vi "Test Tree.vi"() -> ()   [LabVIEW 2020]
uses:
  <vilib>/ActorFramework/Actor/Actor.lvclass
  Views/System Tree View/System Tree View/[V]System Tree View.lvclass
  Depden On/Abstruct View/Abstruct View Messages/Insert Panel Msg/Insert Panel Msg.lvclass
  <vilib>/ActorFramework/Stop Msg/Stop Msg.lvclass
  C:/Program Files (x86)/National Instruments/LabVIEW 2020/vi.lib/ActorFramework/Actor/Actor.lvclass
panel:
  out "NewVal":string[](array[string])
  in  "Tree":string[](tree)
  in  "Stop":bool
  out "error out":errorcluster
  # "LanuncherTree"
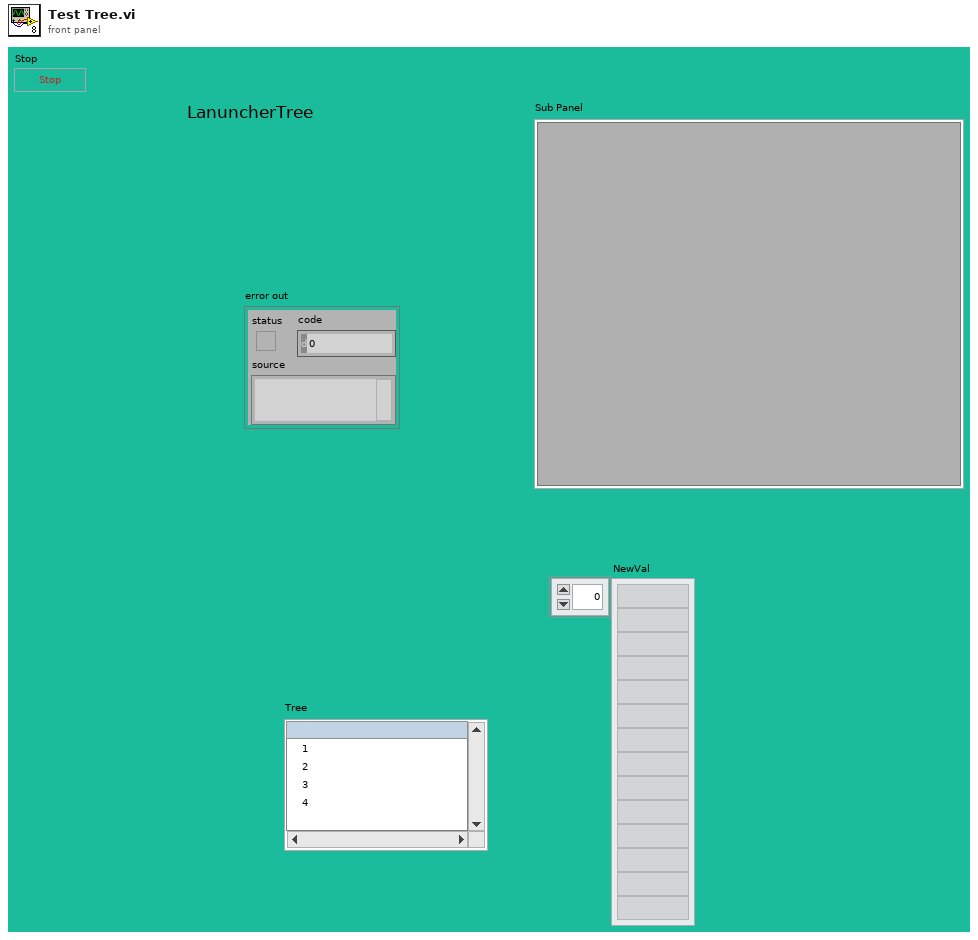
[diagram p1: front panel]
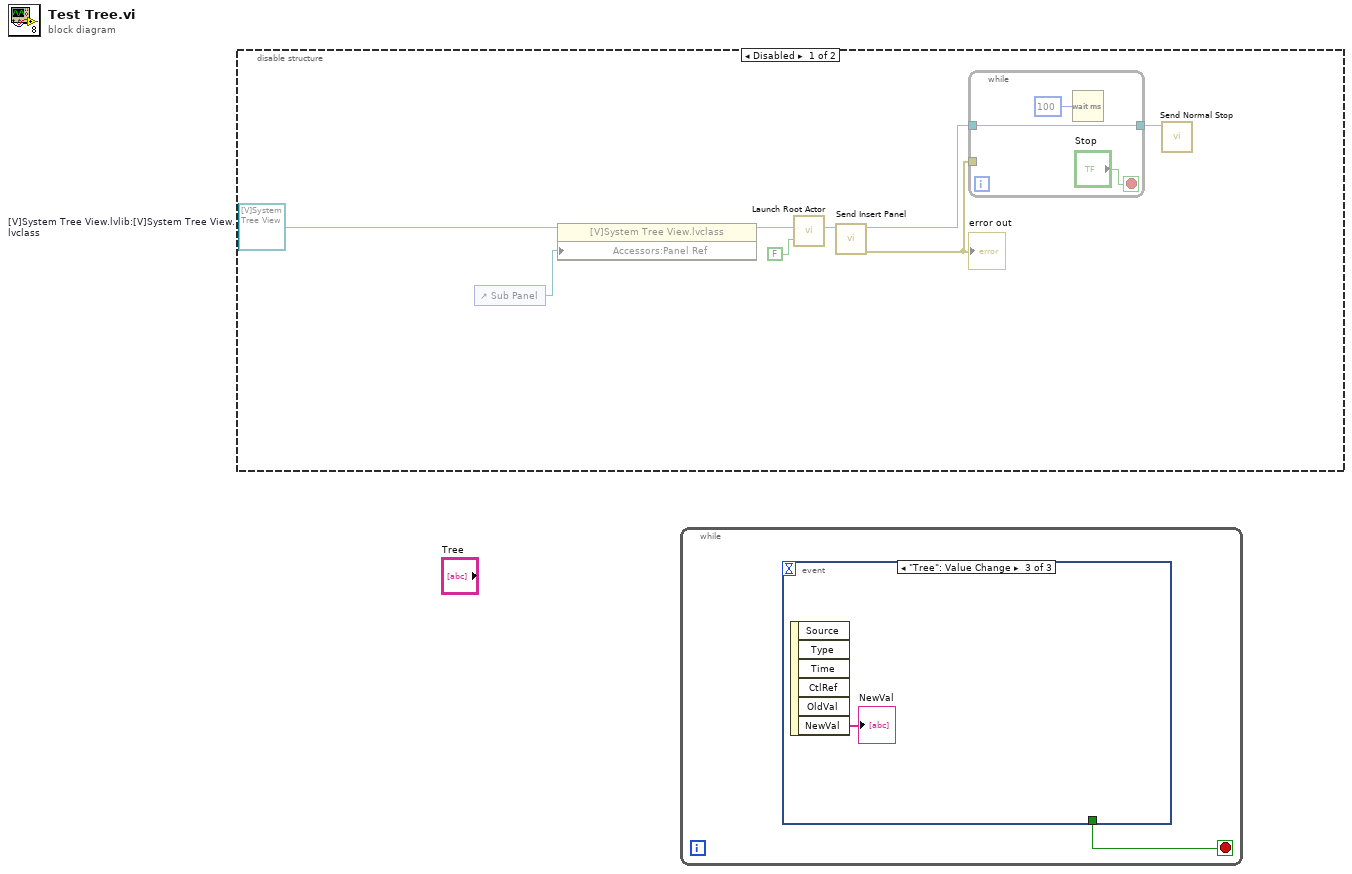
[diagram p0: block diagram]
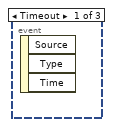
[diagram p2: hidden frame]
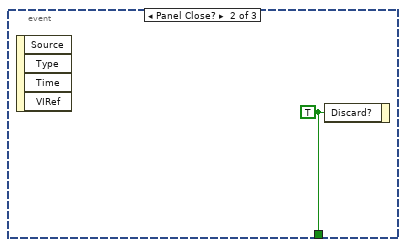
[diagram p3: hidden frame]
diagram:
  n1 = disable-structure shown="Disabled" {
    frame Disabled {
      w7 = refnum<class "[V]System Tree View.lvclass"> refnum  # [V]System Tree View.lvlib:[V]System Tree View.lvclass
      n2 = control-ref of="Sub Panel"() -> (w4:refnum<vi>)
      n3 = property class="[V]System Tree View.lvclass"(reference=w7, "Accessors:Panel Ref"=w4) -> (reference out=w6:refnum<class "[V]System Tree View.lvclass">)  [unwired: 1 in, 1 out]
      n4 = call <vilib>:"Launch Root Actor.vi"("Open Actor Core front panel? (F)"=FALSE, "Actor"=w6) -> ("Actor's Enqueuer"=w3:refnum<class "Message Enqueuer.lvclass">)  [unwired: 8 in, 1 out]
      n5 = call "Send Insert Panel.vi"("Message Enqueuer"=w3) -> ("error out"=w5:errorcluster, "Message Enqueuer out"=w2:refnum<class "Message Enqueuer.lvclass">)  [unwired: 9 in]
      "error out" <- w5
      n6 = while {
        tunnel: w5 -> [_]
        tunnel: w2 -> [w9]
        tunnel: [w9] -> w1
        stop <- "Stop" stop-if-true
        n7 = Wait (ms)(milliseconds to wait=u32 100) -> ()  [unwired: 1 out]
      }
      n8 = call <vilib>:"Send Normal Stop.vi"("Message Enqueuer"=w1) -> ()  [unwired: 10 in, 1 out]
    }
    frame Enabled {
    }
  }
  n9 = while {
    stop <- w12 stop-if-true
    n10 = event shown="[2] \"Tree\": Value Change" {
      selector: _ -> [_ _ _]
      dyn-events: _ -> [_ _ _]
      timeout: _ -> [_ _ _]
      tunnel: [_ w13 _] -> w12
      event Timeout {
        n11 = event-data() -> ()  [unwired: 1 in, 3 out]
      }
      event Panel Close? {
        w13 = TRUE ("Discard?")
        n12 = event-data() -> ()  [unwired: 1 in, 4 out]
        n13 = event-data("Discard?"=w13) -> ()  [unwired: 1 in, 1 out]
      }
      event "Tree": Value Change {
        n14 = event-data() -> ("NewVal"=→"NewVal":string[])  [unwired: 1 in, 5 out]
      }
    }
  }
